vi "NotifyIcon - .NET EventCallback.vi"(4 "Variant":variant, 5 "Event Data":cluster{"sender":refnum<k24>, "e":refnum<k24>}, 6 "Control Ref":refnum<k24>, 7 "Event Common Data":T1) -> ()   [LabVIEW 2009]
uses:
  TypeDefs/NotifyIcon .NET Callback Parameter.ctl
  TypeDefs/NotifyIcon User Event Ref.ctl
  TypeDefs/NotifyIcon Event Data.ctl
  TypeDefs/NotifyIcon Events.ctl
  System.Windows.Forms
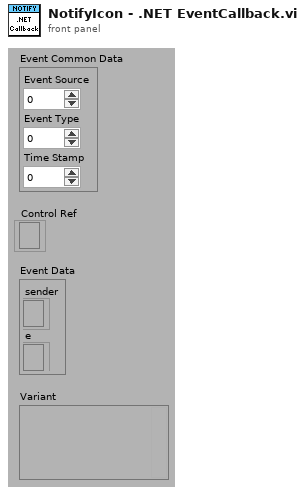
[diagram p1: front panel]
types:
  T1 = cluster{"Event Source":i32, "Event Type":u32, "Time Stamp":u32}
  T2 = typedef "NotifyIcon Events.ctl" = enum16{"BalloonTipClicked", "BalloonTipClosed", "BalloonTipShown", "Click", "Disposed", "DoubleClick", "MouseClick", "MouseDoubleClick", "MouseDown", "MouseMove", "MouseUp", "MenuItemClick", "MenuItemSelect"}
  T3 = typedef "NotifyIcon Event Data.ctl" = cluster{"NotifyIcon Event":T2, "Data String":string}
  T4 = typedef "NotifyIcon .NET Callback Parameter.ctl" = cluster{"NotifyIcon User Event Ref":T5, "Event Data":variant}
  T5 = typedef "NotifyIcon User Event Ref.ctl" = refnum<user-event>
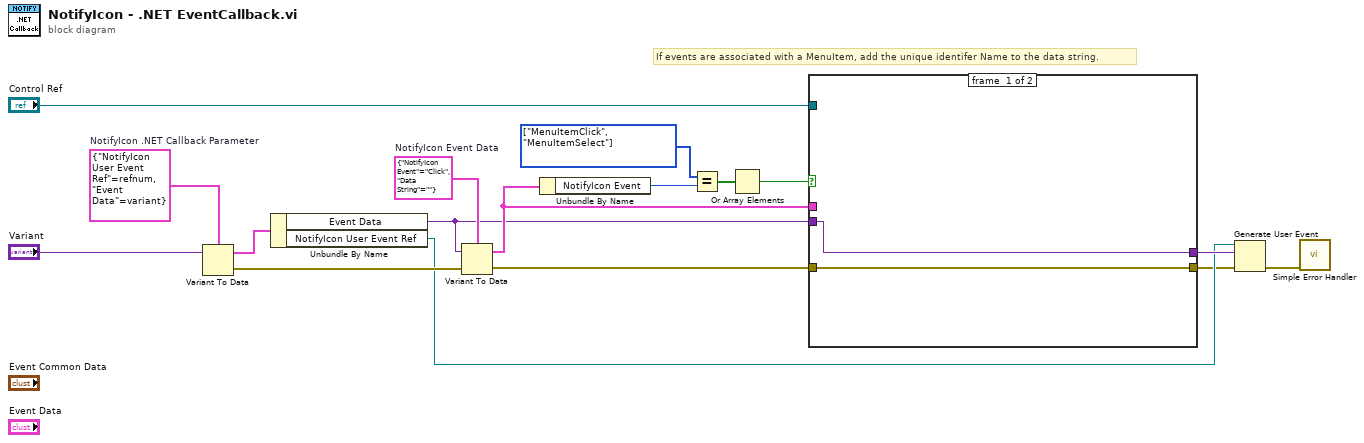
[diagram p0: block diagram]
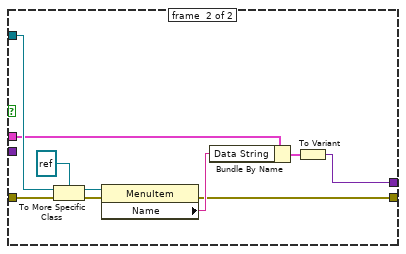
[diagram p2: hidden frame]
diagram:
  w11 = T2[] [enum."MenuItemClick", enum."MenuItemSelect"] items=["BalloonTipClicked", "BalloonTipClosed", "BalloonTipShown", "Click", "Disposed", "DoubleClick", "MouseClick", "MouseDoubleClick", "MouseDown", "MouseMove", "MouseUp", "MenuItemClick", "MenuItemSelect"]
  w13 = T3 {"NotifyIcon Event"=enum."Click", "Data String"=""}  # NotifyIcon Event Data
  w14 = T4 {"NotifyIcon User Event Ref"=refnum, "Event Data"=variant}  # NotifyIcon .NET Callback Parameter
  # "If events are associated with a MenuItem, add the unique identifer Name to the data string."
  n1 = Variant To Data(Variant="Variant", type=w14) -> (error out=w7:errorcluster, data=w15:T4)  [unwired: 1 in]
  n2 = Unbundle By Name(w15) -> ("Event Data"=w3:variant, "NotifyIcon User Event Ref"=w2:T5)
  n3 = Variant To Data(error in=w7, Variant=w3, type=w13) -> (error out=w6:errorcluster, data=w5:T3)
  n4 = Unbundle By Name(w5) -> ("NotifyIcon Event"=w12:T2)
  n5 = Equal?(x=w11, y=w12) -> (x = y?=w10:bool[])
  n6 = Or Array Elements(Boolean array=w10) -> (logical OR=w9:bool)
  n7 = case shown="True" w9 {
    tunnel: "Control Ref" -> [_ w28]
    tunnel: w6 -> [w18 w27]
    tunnel: w5 -> [_ w24]
    tunnel: [w19 w21] -> w4
    tunnel: w3 -> [w19 _]
    tunnel: [w18 w20] -> w1
    frame #0 {
    }
    frame #1 {
      n8 = To More Specific Class(target class=refnum<k24> refnum ("reference"), reference=w28, error in=w27) -> (specific class reference=w26:refnum<k24>, error out=w25:errorcluster)
      n9 = property class="MenuItem"(reference=w26, error in=w25) -> (error out=w20:errorcluster, "Name"=w23:string)  [unwired: 1 out]
      n10 = Bundle By Name(cluster=w24, "Data String"=w23) -> (w22:T3)
      n11 = To Variant(anything=w22) -> (Variant=w21:variant)
    }
  }
  n12 = Generate User Event(user event=w2, event data cluster=w4, error in=w1) -> (error out=w16:errorcluster)  [unwired: 1 out]
  n13 = call <vilib>:"Simple Error Handler.vi"("error in (no error)"=w16) -> ()  [unwired: 4 in, 5 out]
